vi "Test Motors.vi"() -> ()   [LabVIEW 2013]
uses:
  <vilib>/robotics/Starter Kit/2.0/9632 Host Interface/NI_Robotics_Starter Kit Host_9632_2.0.lvclass
  <vilib>/robotics/Utilities/RPM to Radians per Second (Scalar).vi
  <vilib>/robotics/Utilities/Radians per Second to RPM (Scalar).vi
  <vilib>/robotics/Utilities/NI_Robotics Utilities.lvlib
  <vilib>/robotics/Starter Kit/Host Interface/NI_Robotics_Starter Kit Host.lvclass
panel:
  out "Right Velocity":dbl
  out "Right Setpoint":dbl
  out "Left Velocity":dbl
  out "Left Setpoint":dbl
  in  "Kinect  interface":dbl
  out "Wheel Velocities (rpm)":cluster{"Left":dbl, dbl, "Right":dbl, dbl}(graph)
  in  "stop":bool
  # "基于Kinect的移动机器人设计的Labview程序"
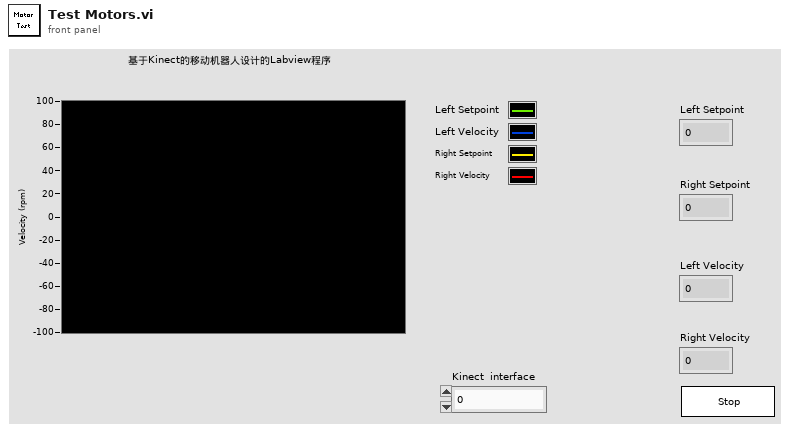
[diagram p1: front panel]
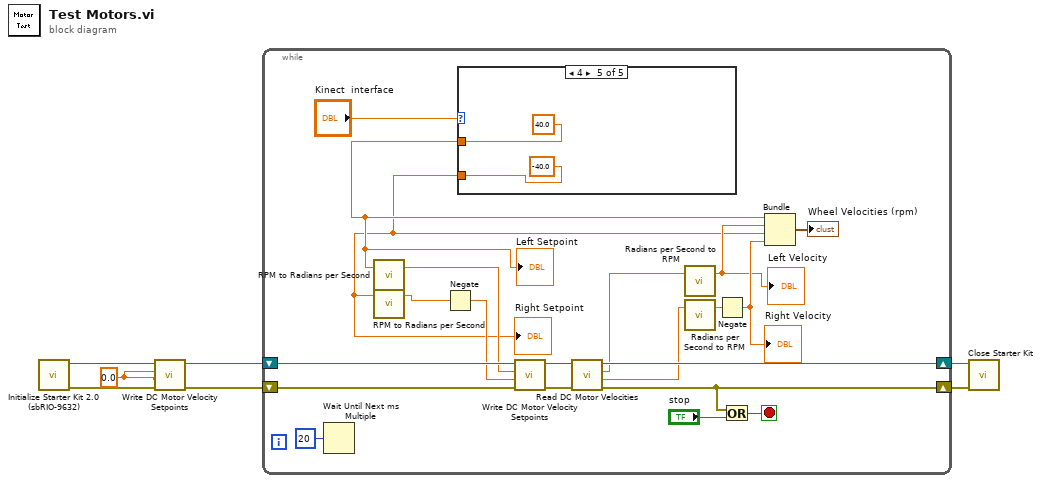
[diagram p0: block diagram]
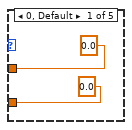
[diagram p2: hidden frame]
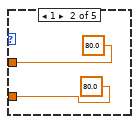
[diagram p3: hidden frame]
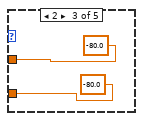
[diagram p4: hidden frame]
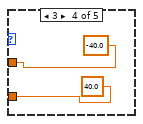
[diagram p5: hidden frame]
diagram:
  w1 = 0.0
  n1 = call <vilib>:"Initialize Starter Kit 2.0 (sbRIO-9632).vi"() -> ("error out"=w3:errorcluster, "FPGA starter kit host 2.0 out"=w2:refnum<class "NI_Robotics_Starter Kit Host_9632_2.0.lvclass">)  [unwired: 10 in]
  n2 = call <vilib>:"Write DC Motor Velocity Setpoints.vi"("error in (no error)"=w3, "right motor ccw velocity (rad/s)"=w1, "left motor ccw velocity (rad/s)"=w1, "starter kit host in"=w2) -> ("error out"=w6:errorcluster, "starter kit host out"=w7:refnum<class "NI_Robotics_Starter Kit Host_9632_2.0.lvclass">)  [unwired: 6 in]
  n3 = while {
    shift-right: [w18] -> w4
    shift-left: w6 -> [w22]
    shift-right: [w19] -> w5
    shift-left: w7 -> [w23]
    stop <- w28 stop-if-true
    n4 = Wait Until Next ms Multiple(millisecond multiple=u32 20) -> ()  [unwired: 1 out]
    n5 = case shown="4" "Kinect  interface" {
      tunnel: [0.0 80.0 -80.0 -40.0 40.0] -> w9
      tunnel: [0.0 80.0 -80.0 40.0 -40.0] -> w8
      frame 0, Default {
      }
      frame 1 {
      }
      frame 2 {
      }
      frame 3 {
      }
      frame 4 {
      }
    }
    "Left Setpoint" <- w9
    "Right Setpoint" <- w8
    n6 = call-poly <vilib>:"RPM to Radians per Second.vi"("rpm"=w9) -> ("radians per second"=w12:dbl)  [unwired: 2 in]
    n7 = call-poly <vilib>:"RPM to Radians per Second.vi"("rpm"=w8) -> ("radians per second"=w16:dbl)  [unwired: 2 in]
    n8 = Negate(x=w16) -> (-x=w13:dbl)
    n9 = call <vilib>:"Write DC Motor Velocity Setpoints.vi"("error in (no error)"=w22, "right motor ccw velocity (rad/s)"=w13, "left motor ccw velocity (rad/s)"=w12, "starter kit host in"=w23) -> ("error out"=w20:errorcluster, "starter kit host out"=w21:refnum<class "NI_Robotics_Starter Kit Host_9632_2.0.lvclass">)  [unwired: 6 in]
    n10 = call <vilib>:"Read DC Motor Velocities.vi"("error in (no error)"=w20, "starter kit host in"=w21) -> ("error out"=w18:errorcluster, "right motor ccw velocity (rad/s)"=w14:dbl, "left motor ccw velocity (rad/s)"=w15:dbl, "starter kit host out"=w19:refnum<class "NI_Robotics_Starter Kit Host_9632_2.0.lvclass">)  [unwired: 6 in]
    n11 = call-poly <vilib>:"Radians per Second to RPM.vi"("radians per second"=w15) -> ("rpm"=w10:dbl)  [unwired: 2 in]
    "Left Velocity" <- w10
    n12 = call-poly <vilib>:"Radians per Second to RPM.vi"("radians per second"=w14) -> ("rpm"=w25:dbl)  [unwired: 2 in]
    n13 = Negate(x=w25) -> (-x=w11:dbl)
    "Right Velocity" <- w11
    n14 = Or(x=w18, y="stop") -> (x .or. y?=w28:bool)
    n15 = Bundle(w9, "rpm"=w10, w8, w11) -> (→"Wheel Velocities (rpm)":cluster{dbl, "rpm":dbl, dbl, dbl})  [unwired: 1 in]
  }
  n16 = call-dynamic "Close Starter Kit.vi"("error in (no error)"=w4, "starter kit host in"=w5) -> ()  [unwired: 9 in, 1 out]
